vi "GetBdcst.vi"(8 "ErrorArray":errorcluster[](array[cluster]), 9 "BdcstInfo":variant, 11 "Test.lvclass":refnum<class "Test.lvclass">) -> (0 "ErrorArray":errorcluster[](array[cluster]), 3 "Test.lvclass":refnum<class "Test.lvclass">)   [LabVIEW 2014, in "Test.lvclass"]
uses:
  Test.lvclass
  Typedef/BdcstInfo.ctl
  Test.lvclass/Test.ctl
  Sync/SyncModule/Protected/clEventType.ctl
  Digitizer/DigitizerModule/Protected/clEventType.ctl
  Accessors/Read ErrorSeverity.vi
  <vilib>/Utility/error.llb/Error Cluster From Error Code.vi
  <vilib>/ErrorRing/Error Ring.xnode
  <userlib>/NIST/NISTErrorLib/NISTErrorLib.lvlib
  Sync/SyncModule/SyncModule.lvlib
  Digitizer/DigitizerModule/DigitizerModule.lvlib
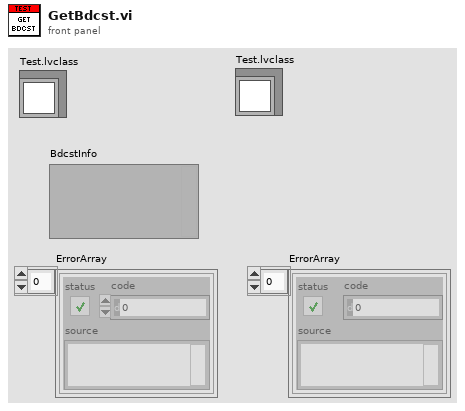
[diagram p1: front panel]
types:
  T1 = typedef "Test.lvclass/BdcstInfo.ctl" = cluster{"ModuleID":i32, "ModuleType":string, "UserEvtRef":variant, "ScriptCmd":string, "Timeout":i32}
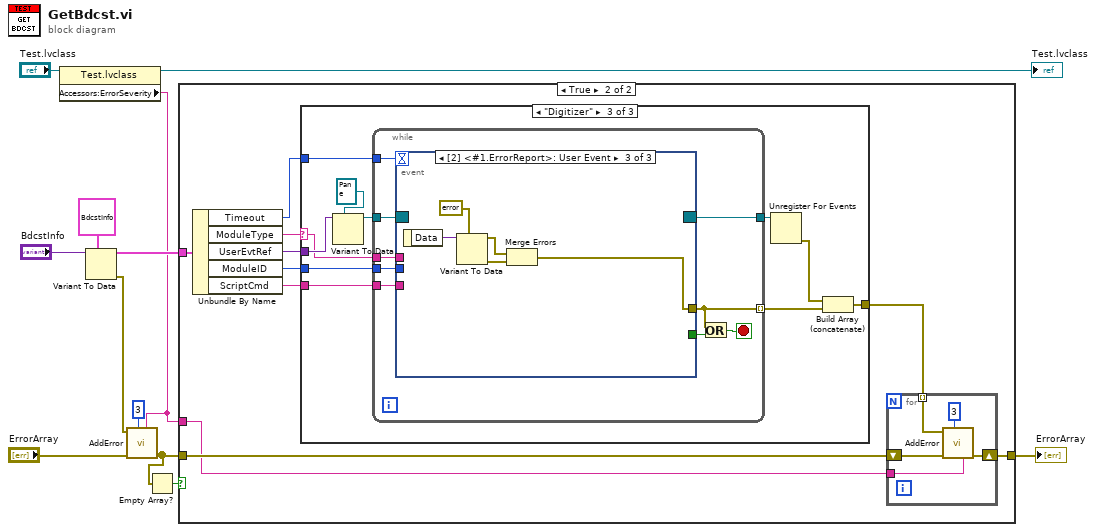
[diagram p0: block diagram]
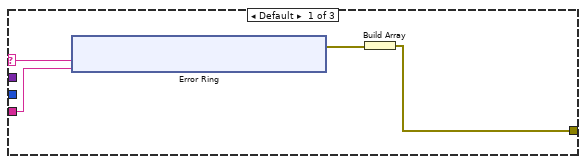
[diagram p3: hidden frame]
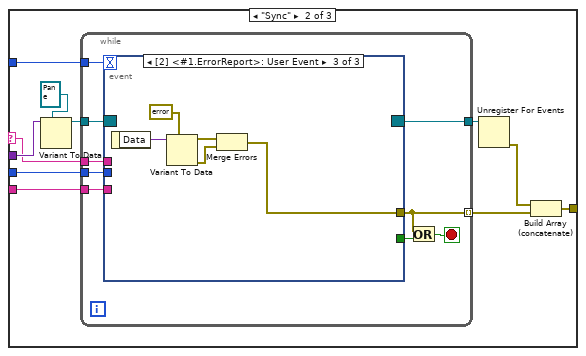
[diagram p4: hidden frame]
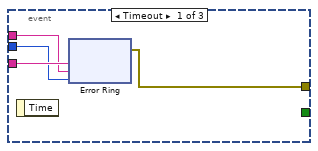
[diagram p5: hidden frame]
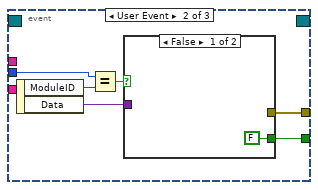
[diagram p6: hidden frame]
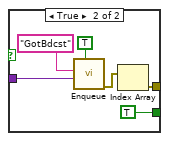
[diagram p7: hidden frame]
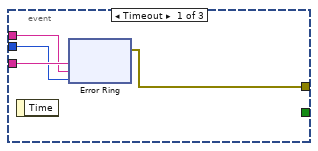
[diagram p8: hidden frame]
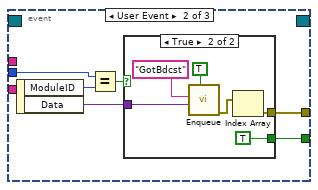
[diagram p9: hidden frame]
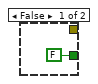
[diagram p10: hidden frame]
diagram:
  n1 = property class="Test.lvclass"(reference="Test.lvclass") -> (reference out=→"Test.lvclass":refnum<class "Test.lvclass">, "Accessors:ErrorSeverity"=w3:string)  [unwired: 1 in, 1 out]
  n2 = Variant To Data(type=T1 {"ModuleID"=0, "ModuleType"="", "UserEvtRef"=variant, "ScriptCmd"="", "Timeout"=5000} ("BdcstInfo"), Variant="BdcstInfo") -> (data=w6:T1, error out=w5:errorcluster)  [unwired: 1 in]
  n3 = call <userlib>:"AddError.vi"("Severity"=w3, "Priority"=u8 3, "ErrorArray"="ErrorArray", "error in (no error)"=w5) -> ("ErrorArray"=w2:errorcluster[])  [unwired: 6 in, 1 out]
  n4 = Empty Array?(array=w2) -> (empty?=w12:bool)
  n5 = case shown="True" w12 {
    tunnel: w2 -> [w13 w20]
    tunnel: [w13 w15] -> w10
    tunnel: w6 -> [_ w23]
    tunnel: w3 -> [_ w19]
    frame False {
    }
    frame True {
      n6 = Unbundle By Name(w23) -> ("Timeout"=w16:i32, "ModuleType"=w22:string, "UserEvtRef"=w18:variant, "ModuleID"=w17:i32, "ScriptCmd"=w21:string)
      n7 = case shown="\"Digitizer\"" w22 {
        selector: w22 -> [w32 w48 w99]
        tunnel: w21 -> [w31 w46 w97]
        tunnel: w18 -> [_ w51 w102]
        tunnel: w17 -> [_ w47 w98]
        tunnel: w16 -> [_ w49 w100]
        tunnel: [w29 w42 w93] -> w14
        frame Default {
          n8 = xnode "Error Ring"("parameter 0"=w32, "parameter 1"=w31) -> ("error out"=w30:errorcluster)
          n9 = Build Array(w30) -> (w29:errorcluster[])
        }
        frame "Sync" {
          n10 = Variant To Data(type=refnum<event-registration> refnum ("Event Registration Refnum"), Variant=w51) -> (data=w50:refnum<event-registration>)  [unwired: 1 in, 1 out]
          n11 = while {
            tunnel: w50 -> [w60]
            tunnel: w49 -> [w59]
            tunnel: w48 -> [w58]
            tunnel: w47 -> [w57]
            tunnel: w46 -> [w56]
            tunnel: [w53] -> w43 mode=indexing
            tunnel: [w52] -> w45
            stop <- w54 stop-if-true
            n12 = event shown="[2] <#1.ErrorReport>: User Event" {
              selector: w60 -> [_ _ _]
              dyn-events: [_ _ _] -> w52
              timeout: w59 -> [_ _ _]
              tunnel: w58 -> [w63 _ _]
              tunnel: w57 -> [w62 w78 _]
              tunnel: w56 -> [w64 _ _]
              tunnel: [w61 w75 w88] -> w53
              tunnel: [_ w74 _] -> w55
              event Timeout {
                n13 = event-data() -> ()  [unwired: 1 in, 1 out]
                n14 = xnode "Error Ring"("parameter 0"=w64, "parameter 1"=w63, "parameter 2"=w62) -> ("error out"=w61:errorcluster)
              }
              event User Event {
                n15 = event-data() -> ("ModuleID"=w79:i32, "Data"=w77:variant)  [unwired: 1 in]
                n16 = Equal?(x=w78, y=w79) -> (x = y?=w76:bool)
                n17 = case shown="False" w76 {
                  tunnel: w77 -> [_ w85]
                  tunnel: [_ w83] -> w75
                  tunnel: [FALSE TRUE] -> w74
                  frame False {
                  }
                  frame True {
                    n18 = call "Enqueue.vi"("Priority? (f)"=TRUE, "Data"=w85, "Message"="GotBdcst") -> ("ErrorArray"=w84:errorcluster[])  [unwired: 8 in]
                    n19 = Index Array(array=w84) -> (element=w83:errorcluster)  [unwired: 1 in]
                  }
                }
              }
              event User Event {
                n20 = event-data() -> ("Data"=w91:variant)  [unwired: 1 in]
                n21 = Variant To Data(type=errorcluster {"status"=FALSE, "code"=0, "source"=""} ("error constant"), Variant=w91) -> (data=w89:errorcluster, error out=w87:errorcluster)  [unwired: 1 in]
                n22 = Merge Errors(w89, w87) -> (w88:errorcluster)
              }
            }
            n23 = Or(x=w53, y=w55) -> (x .or. y?=w54:bool)
          }
          n24 = Unregister For Events(event registration refnum=w45) -> (error out=w44:errorcluster)  [unwired: 1 in]
          n25 = Build Array (concatenate)(w44, w43) -> (w42:errorcluster[])
        }
        frame "Digitizer" {
          n26 = Variant To Data(type=refnum<event-registration> refnum ("Event Registration Refnum"), Variant=w102) -> (data=w101:refnum<event-registration>)  [unwired: 1 in, 1 out]
          n27 = while {
            tunnel: w101 -> [w111]
            tunnel: w100 -> [w110]
            tunnel: w99 -> [w109]
            tunnel: w98 -> [w108]
            tunnel: w97 -> [w107]
            tunnel: [w104] -> w94 mode=indexing
            tunnel: [w103] -> w96
            stop <- w105 stop-if-true
            n28 = event shown="[2] <#1.ErrorReport>: User Event" {
              selector: w111 -> [_ _ _]
              dyn-events: [_ _ _] -> w103
              timeout: w110 -> [_ _ _]
              tunnel: w109 -> [w114 _ _]
              tunnel: w108 -> [w113 w129 _]
              tunnel: w107 -> [w115 _ _]
              tunnel: [w112 w126 w138] -> w104
              tunnel: [_ w125 _] -> w106
              event Timeout {
                n29 = event-data() -> ()  [unwired: 1 in, 1 out]
                n30 = xnode "Error Ring"("parameter 0"=w115, "parameter 1"=w114, "parameter 2"=w113) -> ("error out"=w112:errorcluster)
              }
              event User Event {
                n31 = event-data() -> ("ModuleID"=w130:i32, "Data"=w128:variant)  [unwired: 1 in]
                n32 = Equal?(x=w129, y=w130) -> (x = y?=w127:bool)
                n33 = case shown="True" w127 {
                  tunnel: w128 -> [_ w136]
                  tunnel: [_ w134] -> w126
                  tunnel: [FALSE TRUE] -> w125
                  frame False {
                  }
                  frame True {
                    n34 = call "Enqueue.vi"("Priority? (f)"=TRUE, "Data"=w136, "Message"="GotBdcst") -> ("ErrorArray"=w135:errorcluster[])  [unwired: 8 in]
                    n35 = Index Array(array=w135) -> (element=w134:errorcluster)  [unwired: 1 in]
                  }
                }
              }
              event User Event {
                n36 = event-data() -> ("Data"=w142:variant)  [unwired: 1 in]
                n37 = Variant To Data(type=errorcluster {"status"=FALSE, "code"=0, "source"=""} ("error constant"), Variant=w142) -> (data=w139:errorcluster, error out=w140:errorcluster)  [unwired: 1 in]
                n38 = Merge Errors(w139, w140) -> (w138:errorcluster)
              }
            }
            n39 = Or(x=w104, y=w106) -> (x .or. y?=w105:bool)
          }
          n40 = Unregister For Events(event registration refnum=w96) -> (error out=w95:errorcluster)  [unwired: 1 in]
          n41 = Build Array (concatenate)(w95, w94) -> (w93:errorcluster[])
        }
      }
      n42 = for {
        shift-right: [w28] -> w15
        shift-left: w20 -> [w25]
        tunnel: w19 -> [w27]
        tunnel: w14 -> [w24] mode=indexing
        n43 = call <userlib>:"AddError.vi"("Severity"=w27, "Priority"=u8 3, "ErrorArray"=w25, "error in (no error)"=w24) -> ("ErrorArray"=w28:errorcluster[])  [unwired: 6 in, 1 out]
      }
    }
  }
  "ErrorArray" <- w10
